vi "Pre Launch Init.vi"(11 "Device DDS Communications in":refnum<class "Device DDS Communications.lvclass">) -> (0 "error out":errorcluster, 3 "Device DDS Communications out":refnum<class "Device DDS Communications.lvclass">)   [LabVIEW 2018, in "Device DDS Communications Framework.lvlib" / "Device DDS Communications.lvclass"]
doc: "(<B>Filename</B>: Actor Framework.lvlib:Actor.lvclass:Pre Launch Init.vi)\n\nDefines behavior that occurs after the Launch Nested Actor method is invoked but before the actor's Actor Core method begins running.\n\nBy default, this method does nothing. A descendant class may override it to define behavior."
uses:
  Device DDS Communications.lvclass
  Device DDS Communications.lvclass/Device DDS Communications.ctl
  Device Communication and Control Abstract Actor/Device Communication and Control Abstract/Device Communication and Control Abstract.lvclass
  <vilib>/ORNL/CSEISMIC DDS/DDS Writer/DDS Writer.lvclass
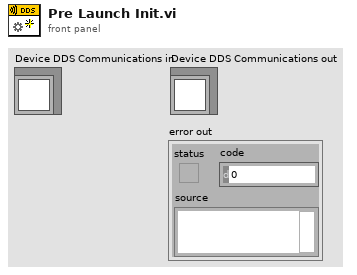
[diagram p1: front panel]
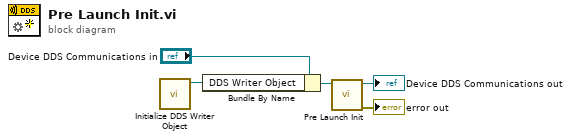
[diagram p0: block diagram]
diagram:
  n1 = call <vilib>:"Initialize DDS Writer Object.vi"() -> ("DDS Writer out"=w1:refnum<class "DDS Writer.lvclass">)  [unwired: 10 in, 1 out]
  n2 = Bundle By Name(cluster="Device DDS Communications in", "DDS Writer Object"=w1) -> (w2:refnum<class "Device DDS Communications.lvclass">)
  n3 = call-parent "Pre Launch Init.vi"("EMS Generic in"=w2) -> ("error out"=→"error out":errorcluster, "EMS Generic out"=→"Device DDS Communications out":refnum<class "Device DDS Communications.lvclass">)  [unwired: 9 in]
